vi "ApplyLayoutToObject.vi"(5 "scaling settings":T1={"scaling factor"={"horizontal"=1.0, "vertical"=1.0}, "scaling to ignore"=variant} {"scaling factor"."vertical" min=0.0; "scaling factor"."horizontal" min=0.0}, 7 "properties to ignore":variant, 8 "error in (no error)":errorcluster, 10 "GObj Refnum":refnum<vi>, 11 "Decoration Layout in":refnum<class "Decoration Layout.lvclass">) -> (0 "error out":errorcluster, 3 "Decoration Layout out":refnum<class "Decoration Layout.lvclass">)   [LabVIEW 2010, in "NI_SE_Front Panel Layout.lvlib" / "Decoration Layout.lvclass"]
doc: "Apply layout information to the GObj Refnum."
uses:
  Decoration Layout.lvclass
  Scaling Factor_Options.ctl
  XY Scaling Factor.ctl
  Object Layout/Object Layout.lvclass
  Decoration Layout.lvclass/Decoration Layout.ctl
  Properties To Ignore.vi
  NI_SE_Front Panel Layout.lvlib
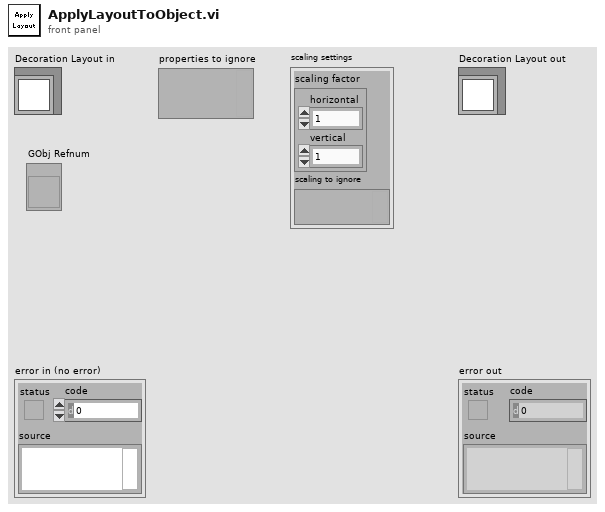
[diagram p1: front panel]
types:
  T1 = typedef "NI_SE_Front Panel Layout.lvlib/Scaling Factor_Options.ctl" = cluster{"scaling factor":T2, "scaling to ignore":variant}
  T2 = typedef "NI_SE_Front Panel Layout.lvlib/XY Scaling Factor.ctl" = cluster{"horizontal":dbl, "vertical":dbl}
  T3 = typedef "LVBoundsTypeDef.ctl" = cluster{"Width":u32, "Height":u32}
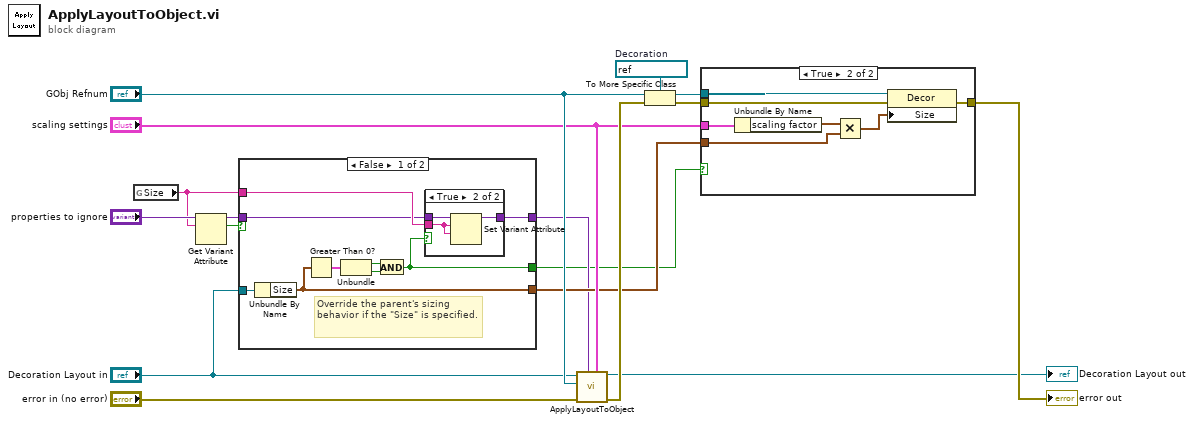
[diagram p0: block diagram]
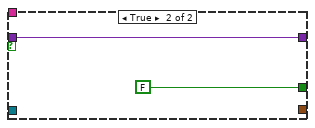
[diagram p3: hidden frame]
diagram:
  w9 = refnum<vi> refnum  # Decoration
  n1 = global read "Properties To Ignore.vi" "Size"() -> (w1:string)
  n2 = Get Variant Attribute(Variant="properties to ignore", name=w1) -> (duplicate Variant=w4:variant, found=w3:bool)  [unwired: 2 in, 2 out]
  n3 = case shown="False" w3 {
    tunnel: "Decoration Layout in" -> [w26 _]
    tunnel: [w22 _] -> w10
    tunnel: [w21 w32] -> w6
    tunnel: w1 -> [w20 _]
    tunnel: w4 -> [w19 w32]
    tunnel: [w18 FALSE] -> w2
    frame False {
      # "Override the parent's sizing behavior if the \"Size\" is specified."
      n4 = Unbundle By Name(w26) -> ("Size"=w22:T3)
      n5 = Greater Than 0?(x=w22) -> (x > 0?=w25:cluster{"Width":bool, "Height":bool})
      n6 = Unbundle(w25) -> ("Width"=w24:bool, "Height"=w23:bool)
      n7 = And(x=w24, y=w23) -> (x .and. y?=w18:bool)
      n8 = case shown="True" w18 {
        tunnel: w19 -> [w27 w30]
        tunnel: [w27 w29] -> w21
        tunnel: w20 -> [_ w28]
        frame False {
        }
        frame True {
          n9 = Set Variant Attribute(Variant=w30, name=w28, value=w28) -> (Variant out=w29:variant)  [unwired: 1 in, 2 out]
        }
      }
    }
    frame True {
    }
  }
  n10 = call-parent "ApplyLayoutToObject.vi"("scaling settings"="scaling settings", "properties to ignore"=w6, "error in (no error)"="error in (no error)", "GObj Refnum"="GObj Refnum", "Object Layout in"="Decoration Layout in") -> ("error out"=w16:errorcluster, "Object Layout out"=→"Decoration Layout out":refnum<class "Decoration Layout.lvclass">)  [unwired: 5 in]
  n11 = To More Specific Class(target class=w9, reference="GObj Refnum", error in=w16) -> (specific class reference=w8:refnum<vi>, error out=w7:errorcluster)
  n12 = case shown="True" w2 {
    tunnel: "scaling settings" -> [_ w40]
    tunnel: w8 -> [_ w38]
    tunnel: w7 -> [w33 w37]
    tunnel: [w33 w35] -> w15
    tunnel: w10 -> [_ w34]
    frame False {
    }
    frame True {
      n13 = Unbundle By Name(w40) -> ("scaling factor"=w39:T2)
      n14 = Multiply(x=w39, y=w34) -> (x*y=w36:T2)
      n15 = property class="Decor"(reference=w38, error in=w37, "Size"=w36) -> (error out=w35:errorcluster)  [unwired: 1 out]
    }
  }
  "error out" <- w15
